vi "Fault_ID_Parse_FL24_Dryer.vi"(8 "Enum":enum16{"Sequence", "Table"}(ring), 11 "Numeric":u32) -> (3 "String":string)   [LabVIEW 2016]
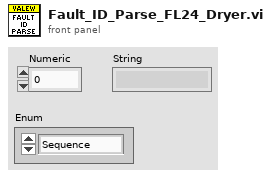
[diagram p1: front panel]
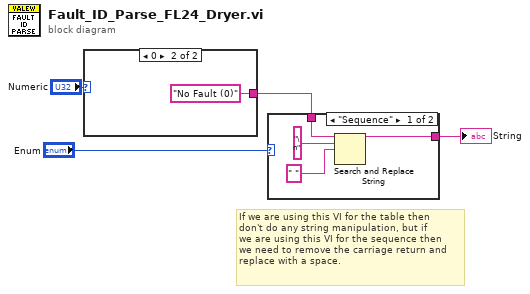
[diagram p0: block diagram]
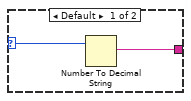
[diagram p3: hidden frame]
diagram:
  # "If we are using this VI for the table then\ndon't do any string manipulation, but if\nwe are using this VI for the sequence then\nwe need to remove the carriage return and\nreplace with a space."
  n1 = case shown="0" "Numeric" {
    selector: "Numeric" -> [w6 _]
    tunnel: [w5 "No Fault (0)"] -> w3
    frame Default {
      n2 = Number To Decimal String(number=w6) -> (decimal integer string=w5:string)  [unwired: 1 in]
    }
    frame 0 {
    }
  }
  n3 = case shown="\"Sequence\"" "Enum" {
    tunnel: w3 -> [w11 w12]
    tunnel: [w8 w12] -> w2
    frame "Sequence" {
      n4 = Search and Replace String(input string=w11, search string="\n", replace string=" " ("replace string (\"\")")) -> (result string=w8:string)  [unwired: 5 in, 3 out]
    }
    frame "Table" {
    }
  }
  "String" <- w2
